vi "Add Port RTM.vi"(8 "error in":errorcluster, 11 "Node Ptr":T3 format="%.0x") -> (0 "error out":errorcluster)   [LabVIEW 2020, in "Communication Bus Template System Explorer.lvlib" / "Implementation.lvlib"]
doc: "This VI runs when the Add Port run-time menu is chosen. It allows the user to create a port with an associated database."
uses:
  Implementation.lvlib
  <vilib>/NI VeriStand/Custom Device API/Custom Device Item Ref.ctl
  Types/XNET Interface Name.ctl
  Types/CAN Cluster.ctl
  Types/Add Port RTM Properties.ctl
  Types/Port Properties.ctl
  Types/Database.ctl
  Types/Frame.ctl
  Types/Signal.ctl
  Types/ECU.ctl
  Scripting/Constants.vi
  <vilib>/NI VeriStand/Custom Device Tools/Custom Device Utility Library/Custom Device Utility Library.lvlib
  Scripting/Communication Bus Template Scripting.lvlib
  <vilib>/NI VeriStand/Custom Device API/Custom Device API.lvlib
panel:
  in  "CAN Cluster":T1
  in  "XNET Interface Name":T2
  in  "Baud Rate":u32
  in  "XNET Database":string(combo)
  in  "Port Name":string
  in  "Help":bool
  in  "Cancel":bool
  in  "OK":bool
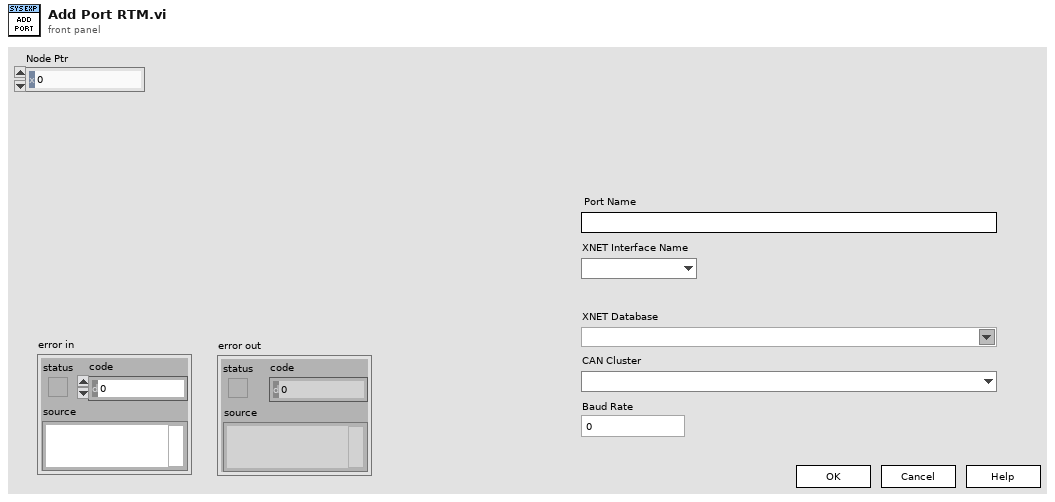
[diagram p1: front panel]
types:
  T1 = typedef "Communication Bus Template System Explorer.lvlib/Implementation.lvlib/CAN Cluster.ctl" = u16
  T2 = typedef "Communication Bus Template System Explorer.lvlib/Implementation.lvlib/XNET Interface Name.ctl" = u16
  T3 = typedef "Custom Device API.lvlib/Custom Device Item Ref.ctl" = u64
  T4 = typedef "Communication Bus Template System Explorer.lvlib/Implementation.lvlib/Add Port RTM Properties.ctl" = cluster{"Port Name":string, "Node Ptr":T3, "Port Properties":T5, "Database":T6[]}
  T5 = typedef "Communication Bus Template System Explorer.lvlib/Implementation.lvlib/Port Properties.ctl" = cluster{"Database Name":string, "Database Path":path, "Baud Rate":u32, "CAN Interface Number":u16, "CAN Cluster":string}
  T6 = typedef "Communication Bus Template System Explorer.lvlib/Implementation.lvlib/Database.ctl" = cluster{"Name":string, "Baud Rate":u64, "Frames":T7[], "ECUs":T9[]}
  T7 = typedef "Communication Bus Template System Explorer.lvlib/Implementation.lvlib/Frame.ctl" = cluster{"Name":string, "ID":u32, "Signals":T8[]}
  T8 = typedef "Communication Bus Template System Explorer.lvlib/Implementation.lvlib/Signal.ctl" = string
  T9 = typedef "Communication Bus Template System Explorer.lvlib/Implementation.lvlib/ECU.ctl" = cluster{"Name":string, "Frames Received Indices":u32[], "Frames Transmitted Indices":u32[]}
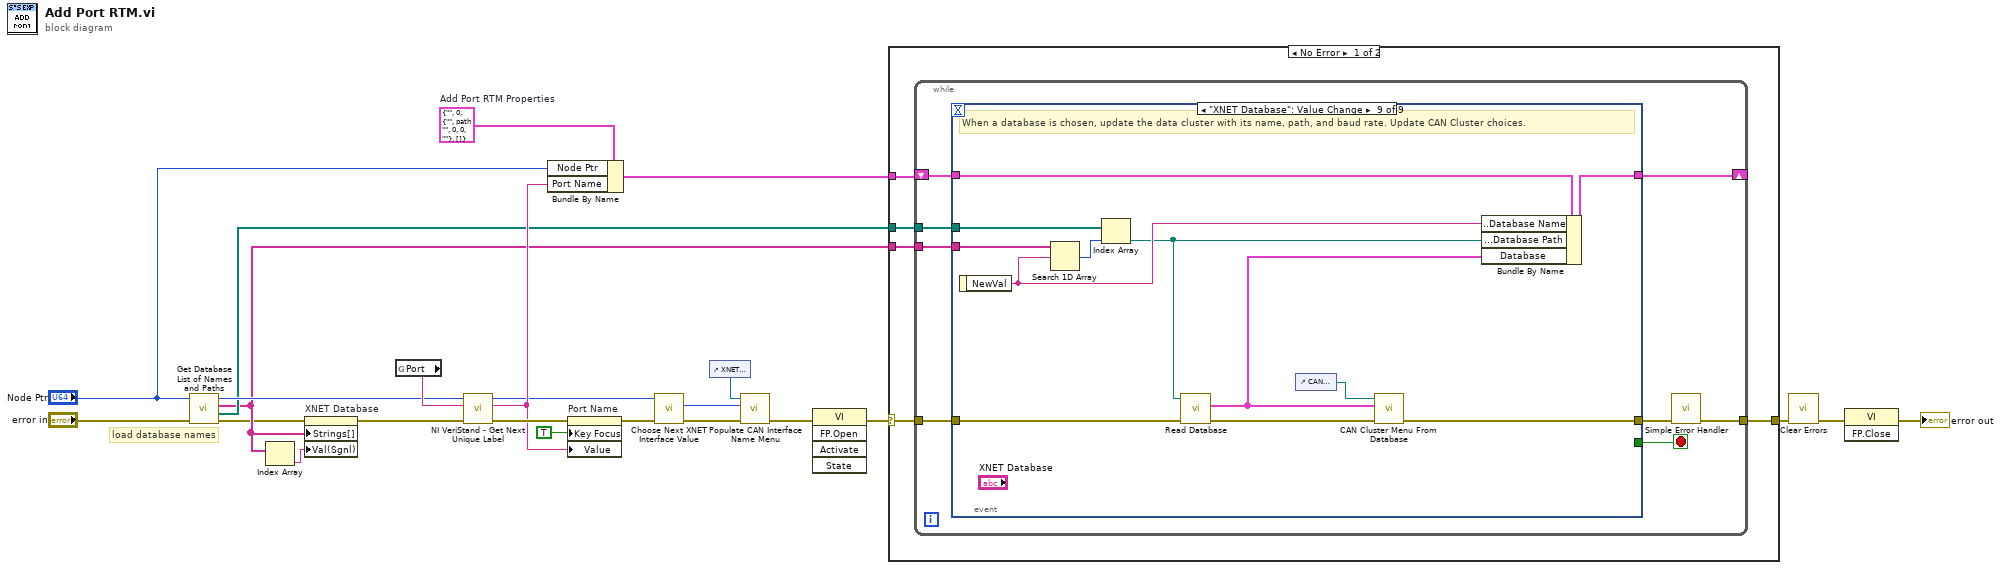
[diagram p0: block diagram]
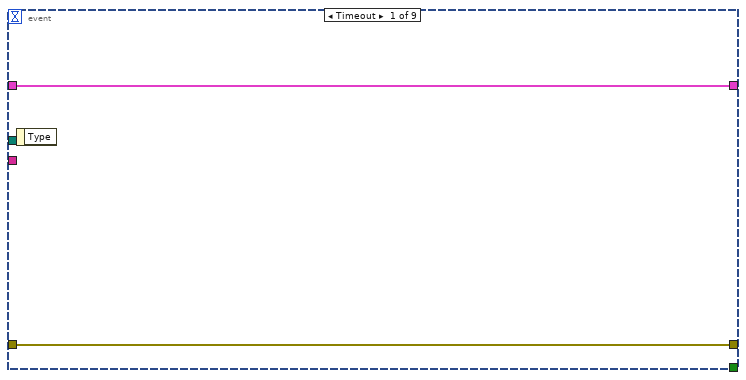
[diagram p2: hidden frame]
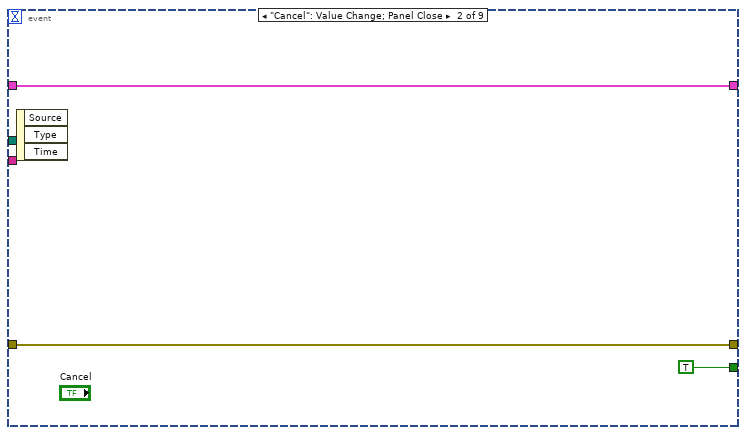
[diagram p3: hidden frame]
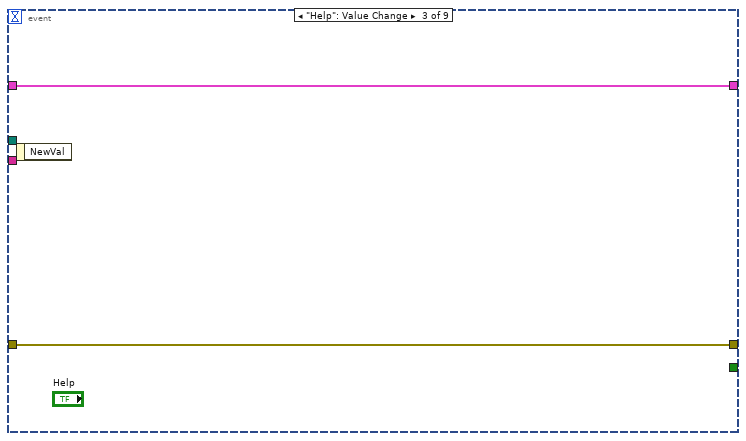
[diagram p4: hidden frame]
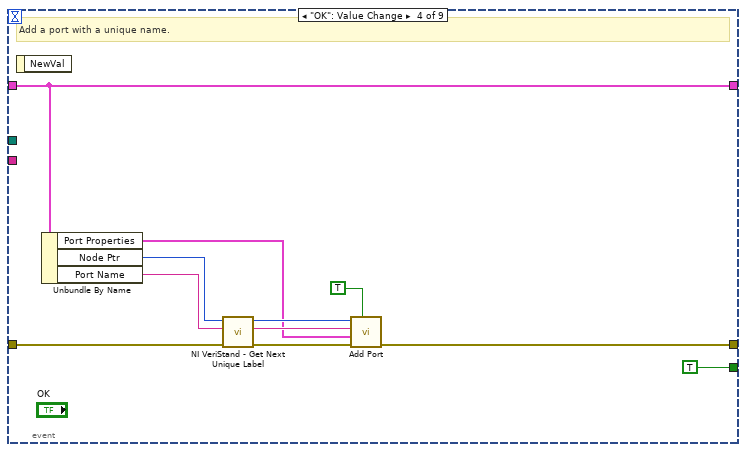
[diagram p5: hidden frame]
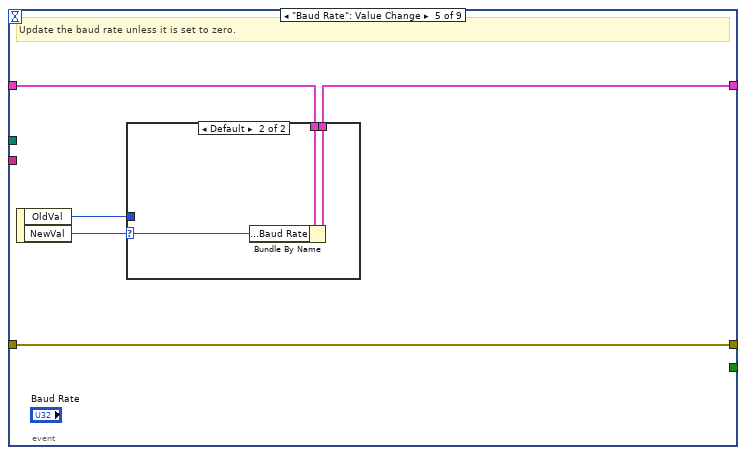
[diagram p6: hidden frame]
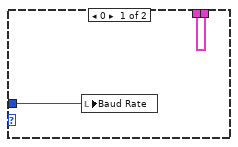
[diagram p7: hidden frame]
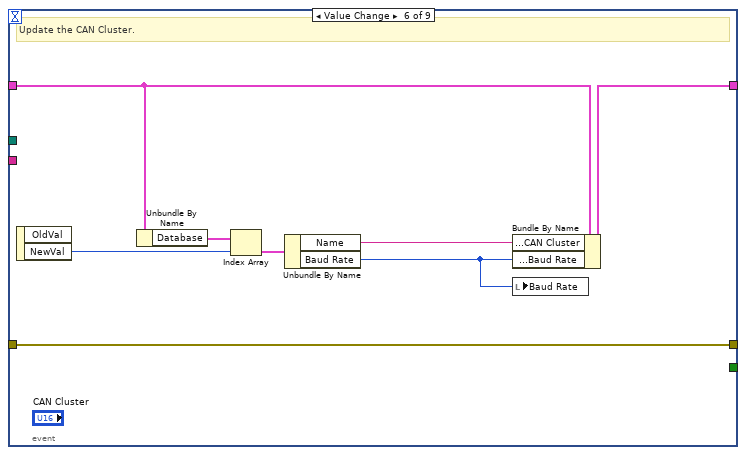
[diagram p8: hidden frame]
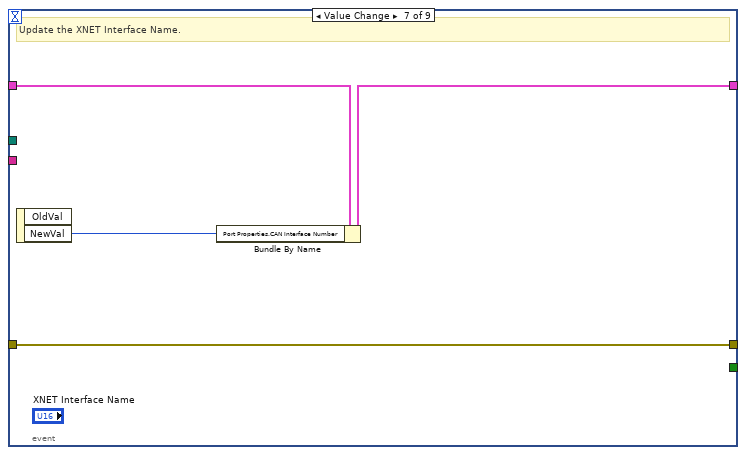
[diagram p9: hidden frame]
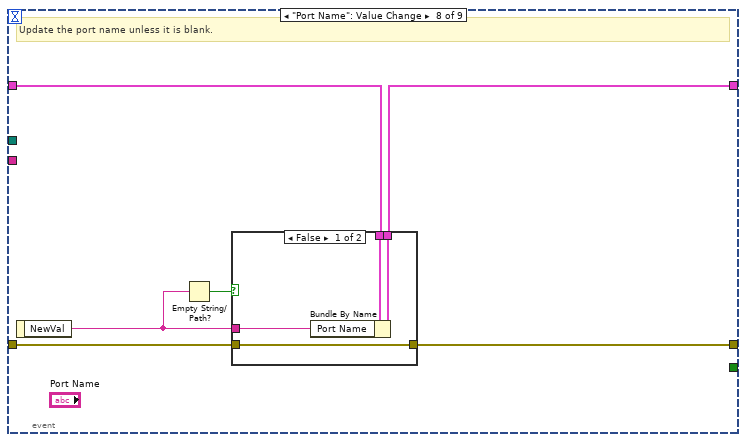
[diagram p10: hidden frame]
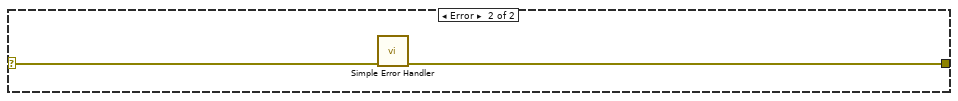
[diagram p12: hidden frame]
diagram:
  w12 = T4 {"Port Name"="", "Node Ptr"=0, "Port Properties"={"Database Name"="", "Database Path"=path "", "Baud Rate"=0, "CAN Interface Number"=0, "CAN Cluster"=""}, "Database"=[]}  # Add Port RTM Properties
  # "load database names"
  n1 = call "Get Database List of Names and Paths.vi"("error in"="error in", "Databases Ref"="Node Ptr") -> ("error out"=w3:errorcluster, "Paths"=w13:path[], "Names"=w8:string[], "Databases Ref out"=w14:T3)  [unwired: 6 in]
  n2 = Index Array(array=w8) -> (element=w9:string)  [unwired: 1 in]
  n3 = property on="XNET Database" class="CmbBox"(error in=w3, "Strings[]"=w8, "Val(Sgnl)"=w9) -> (error out=w2:errorcluster)  [unwired: 1 in, 1 out]
  n4 = global read "Constants.vi" "Port"() -> (w18:string)
  n5 = call <vilib>:"NI VeriStand - Get Next Unique Label.vi"("error in (no error)"=w2, "Label"=w18, "Parent Ref in"=w14) -> ("error out"=w19:errorcluster, "Label out"=w17:string, "Parent Ref dup"=w5:T3)  [unwired: 5 in, 1 out]
  n6 = Bundle By Name(cluster=w12, "Node Ptr"="Node Ptr", "Port Name"=w17) -> (w22:T4)
  n7 = property on="Port Name" class="Str"(error in=w19, "Key Focus"=TRUE, "Value"=w17) -> (error out=w7:errorcluster)  [unwired: 1 in, 1 out]
  n8 = call "Choose Next XNET Interface Value.vi"("error in"=w7, "Databases Ref"=w5) -> ("error out"=w6:errorcluster, "Next Available Value"=w4:u16)  [unwired: 7 in, 1 out]
  n9 = control-ref of="XNET Interface Name"() -> (w10:refnum<vi>)
  n10 = call "Populate CAN Interface Name Menu.vi"("error in"=w6, "Default Value (1)"=w4, "CAN Interface Menu Refnum"=w10) -> ("error out"=w11:errorcluster)  [unwired: 8 in]
  n11 = invoke class="VI" method="FP.Open"(error in=w11) -> (error out=w1:errorcluster)  [unwired: 4 in, 4 out]
  n12 = case shown="No Error" w1 {
    selector: w1 -> [w29 w103]
    tunnel: [w28 w102] -> w23
    tunnel: w22 -> [w27 _]
    tunnel: w8 -> [w26 _]
    tunnel: w13 -> [w25 _]
    frame No Error {
      n13 = while {
        tunnel: w29 -> [w37]
        tunnel: [w35] -> w28
        shift-right: [w32] -> _
        shift-left: w27 -> [w33]
        tunnel: w26 -> [w31]
        tunnel: w25 -> [w30]
        stop <- w34 stop-if-true
        n14 = event shown="[8] \"XNET Database\": Value Change" {
          selector: _ -> [_ _ _ _ _ _ _ _ _]
          dyn-events: _ -> [_ _ _ _ _ _ _ _ _]
          timeout: _ -> [_ _ _ _ _ _ _ _ _]
          tunnel: [w39 w41 w44 w45 w56 w72 w75 w82 w90] -> w36
          tunnel: w37 -> [w39 w41 w44 w54 w56 w72 w75 w83 w94]
          tunnel: [_ TRUE ("Discard?") _ TRUE ("Discard?") _ _ _ _ _] -> w34
          tunnel: w33 -> [w38 w40 w43 w53 w58 w71 w76 w79 w100]
          tunnel: [w38 w40 w43 w53 w59 w73 w77 w78 w101] -> w32
          tunnel: w31 -> [_ _ _ _ _ _ _ _ w97]
          tunnel: w30 -> [_ _ _ _ _ _ _ _ w98]
          event Timeout {
            n15 = event-data() -> ()  [unwired: 1 in, 1 out]
          }
          event "Cancel": Value Change; Panel Close {
            n16 = event-data() -> ()  [unwired: 1 in, 3 out]
          }
          event "Help": Value Change {
            n17 = event-data() -> ()  [unwired: 1 in, 1 out]
          }
          event "OK": Value Change {
            # "Add a port with a unique name."
            n18 = event-data() -> ()  [unwired: 1 in, 1 out]
            n19 = Unbundle By Name(w53) -> ("Port Properties"=w46:T5, "Node Ptr"=w52:T3, "Port Name"=w51:string)
            n20 = call <vilib>:"NI VeriStand - Get Next Unique Label.vi"("error in (no error)"=w54, "Label"=w51, "Parent Ref in"=w52) -> ("error out"=w50:errorcluster, "Label out"=w48:string, "Parent Ref dup"=w49:T3)  [unwired: 5 in, 1 out]
            n21 = call "Add Port.vi"("Highlight? (F)"=TRUE, "error in"=w50, "Port Properties"=w46, "Port Name"=w48, "Ports Ref"=w49) -> ("error out"=w45:errorcluster)  [unwired: 5 in, 1 out]
          }
          event "Baud Rate": Value Change {
            # "Update the baud rate unless it is set to zero."
            n22 = event-data() -> ("OldVal"=w57:u32, "NewVal"=w60:u32)  [unwired: 1 in]
            n23 = case shown="Default" w60 {
              selector: w60 -> [_ w63]
              tunnel: w58 -> [w62 w65]
              tunnel: [w62 w64] -> w59
              tunnel: w57 -> [w61 _]
              frame 0 {
                n24 = local write "Baud Rate"(w61) -> ()
              }
              frame Default {
                n25 = Bundle By Name(cluster=w65, "Port Properties.Baud Rate"=w63) -> (w64:T4)
              }
            }
          }
          event Value Change {
            # "Update the CAN Cluster."
            n26 = event-data() -> ("NewVal"=w69:T1)  [unwired: 1 in, 1 out]
            n27 = Unbundle By Name(w71) -> ("Database"=w70:T6[])
            n28 = Index Array(array=w70, index=w69) -> (element=w68:T6)
            n29 = Unbundle By Name(w68) -> ("Name"=w67:string, "Baud Rate"=w66:u64)
            n30 = Bundle By Name(cluster=w71, "Port Properties.CAN Cluster"=w67, "Port Properties.Baud Rate"=w66) -> (w73:T4)
            n31 = local write "Baud Rate"(w66) -> ()
          }
          event Value Change {
            # "Update the XNET Interface Name."
            n32 = event-data() -> ("NewVal"=w74:T2)  [unwired: 1 in, 1 out]
            n33 = Bundle By Name(cluster=w76, "Port Properties.CAN Interface Number"=w74) -> (w77:T4)
          }
          event "Port Name": Value Change {
            # "Update the port name unless it is blank."
            n34 = event-data() -> ("NewVal"=w80:string)  [unwired: 1 in]
            n35 = Empty String/Path?(string/path=w80) -> (empty?=w81:bool)
            n36 = case shown="False" w81 {
              tunnel: w83 -> [w87 w89]
              tunnel: w80 -> [w85 _]
              tunnel: [w87 w89] -> w82
              tunnel: w79 -> [w86 w88]
              tunnel: [w84 w88] -> w78
              frame False {
                n37 = Bundle By Name(cluster=w86, "Port Name"=w85) -> (w84:T4)
              }
              frame True {
              }
            }
          }
          event "XNET Database": Value Change {
            # "When a database is chosen, update the data cluster with its name, path, and baud rate. Update CAN Cluster choices."
            n38 = event-data() -> ("NewVal"=w96:string)  [unwired: 1 in]
            n39 = Search 1D Array(1D array=w97, element=w96) -> (index of element=w99:i32)  [unwired: 1 in]
            n40 = Index Array(array=w98, index=w99) -> (element=w95:path)
            n41 = call "Read Database.vi"("error in"=w94, "Path"=w95) -> ("error out"=w93:errorcluster, "Database"=w91:T6[])  [unwired: 8 in]
            n42 = control-ref of="CAN Cluster"() -> (w92:refnum<vi>)
            n43 = call "CAN Cluster Menu From Database.vi"("error in"=w93, "Database"=w91, "CAN Cluster Menu Refnum"=w92) -> ("error out"=w90:errorcluster)  [unwired: 8 in]
            n44 = Bundle By Name(cluster=w100, "Port Properties.Database Name"=w96, "Port Properties.Database Path"=w95, "Database"=w91) -> (w101:T4)
          }
        }
        n45 = call <vilib>:"Simple Error Handler.vi"("error in (no error)"=w36) -> ("error out"=w35:errorcluster)  [unwired: 4 in, 4 out]
      }
    }
    frame Error {
      n46 = call <vilib>:"Simple Error Handler.vi"("error in (no error)"=w103) -> ("error out"=w102:errorcluster)  [unwired: 4 in, 4 out]
    }
  }
  n47 = call <vilib>:"Clear Errors.vi"("error in (no error)"=w23) -> ("error out"=w21:errorcluster)  [unwired: 5 in, 1 out]
  n48 = invoke class="VI" method="FP.Close"(error in=w21) -> (error out=→"error out":errorcluster)  [unwired: 2 in, 2 out]
